vi "measure_once.vi"(8 "error in (no error)":errorcluster caption="エラー入力（エラーなし）", 9 "flux constant":T2, 10 "文字送り間隔 (100 ms)":i16=100, 11 "VISAリソース名":refnum<visa-resource-name>) -> (0 "error out":errorcluster caption="エラー出力", 2 "SQUID data":T1, 3 "VISAリソース名 （出力）":refnum<visa-resource-name>)   [LabVIEW 2017]
uses:
  controls/XYZ_Data.ctl
  controls/SQUID_data.ctl
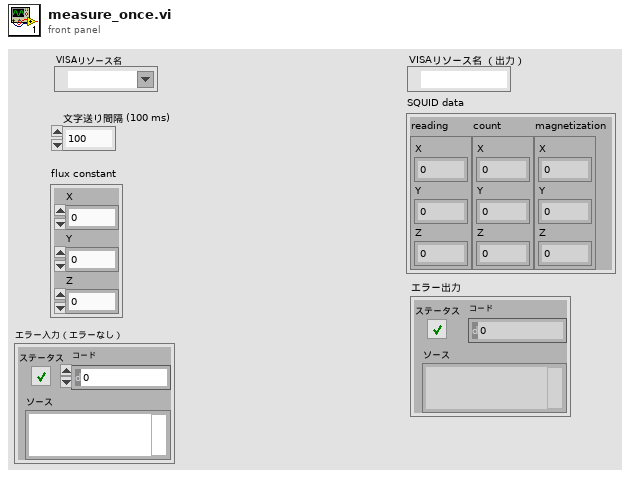
[diagram p1: front panel]
types:
  T1 = typedef "SQUID_data.ctl" = cluster{"reading":T2, "count":T2, "magnetization":T2}
  T2 = typedef "XYZ_Data.ctl" = cluster{"X":dbl, "Y":dbl, "Z":dbl}
  T3 = cluster{"読み取り":string, "読み取り":string, "読み取り":string}
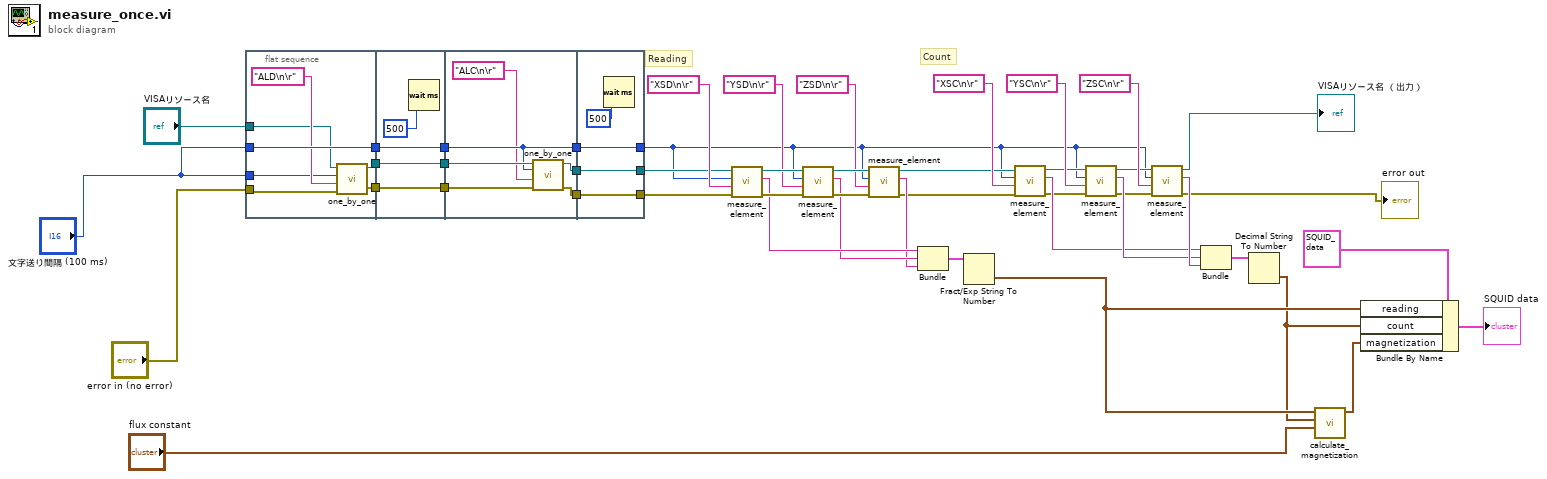
[diagram p0: block diagram]
diagram:
  # "Count"
  # "Reading"
  n1 = flat-sequence {
    tunnel: "文字送り間隔 (100 ms)" -> [w53]
    tunnel: [w48] -> w15
    tunnel: [w53] -> w14
    tunnel: [w49] -> w13
    tunnel: "文字送り間隔 (100 ms)" -> [w51]
    tunnel: "VISAリソース名" -> [w50]
    tunnel: "error in (no error)" -> [w47]
    tunnel: [w57] -> w18
    tunnel: [w55] -> w17
    tunnel: [w56] -> w16
    tunnel: w15 -> [w57]
    tunnel: w14 -> [w55]
    tunnel: w13 -> [w56]
    tunnel: w18 -> [w63]
    tunnel: w17 -> [w58]
    tunnel: w16 -> [w62]
    tunnel: [w61] -> w10
    tunnel: [w59] -> w9
    tunnel: [w58] -> w8
    tunnel: [w66] -> w19
    tunnel: [w67] -> w20
    tunnel: w10 -> [w67]
    tunnel: w9 -> [w66]
    tunnel: [w65] -> _
    tunnel: w8 -> [w65]
    frame #0 {
      n2 = call "one_by_one.vi"("error in (no error)"=w47, "入力文字"="ALD\n\r", "待機 (200ms)"=w51, "VISAリソース名"=w50) -> ("error out"=w49:errorcluster, "VISAリソース名出力"=w48:refnum<visa-resource-name>)  [unwired: 6 in]
    }
    frame #1 {
      n3 = Wait (ms)(milliseconds to wait=500) -> ()  [unwired: 1 out]
    }
    frame #2 {
      n4 = call "one_by_one.vi"("error in (no error)"=w62, "入力文字"="ALC\n\r", "待機 (200ms)"=w58, "VISAリソース名"=w63) -> ("error out"=w61:errorcluster, "VISAリソース名出力"=w59:refnum<visa-resource-name>)  [unwired: 6 in]
    }
    frame #3 {
      n5 = Wait (ms)(milliseconds to wait=500) -> ()  [unwired: 1 out]
    }
  }
  n6 = call "measure_element.vi"("error in (no error)"=w20, "コマンド"="XSD\n\r", "文字送り間隔 (200 ms)"="文字送り間隔 (100 ms)", "VISAリソース名"=w19) -> ("error out"=w44:errorcluster, "読み取り"=w39:string, "VISAリソース名 （出力）"=w45:refnum<visa-resource-name>)  [unwired: 5 in]
  n7 = call "measure_element.vi"("error in (no error)"=w44, "コマンド"="YSD\n\r", "文字送り間隔 (200 ms)"="文字送り間隔 (100 ms)", "VISAリソース名"=w45) -> ("error out"=w42:errorcluster, "読み取り"=w38:string, "VISAリソース名 （出力）"=w43:refnum<visa-resource-name>)  [unwired: 5 in]
  n8 = call "measure_element.vi"("error in (no error)"=w42, "コマンド"="ZSD\n\r", "文字送り間隔 (200 ms)"="文字送り間隔 (100 ms)", "VISAリソース名"=w43) -> ("error out"=w25:errorcluster, "読み取り"=w37:string, "VISAリソース名 （出力）"=w26:refnum<visa-resource-name>)  [unwired: 5 in]
  n9 = Bundle("読み取り"=w39, "読み取り"=w38, "読み取り"=w37) -> (w24:T3)  [unwired: 1 in]
  n10 = Fract/Exp String To Number(string=w24) -> (number=w4:cluster{"読み取り":dbl, "読み取り":dbl, "読み取り":dbl})  [unwired: 3 in, 1 out]
  n11 = call "measure_element.vi"("error in (no error)"=w25, "コマンド"="XSC\n\r", "文字送り間隔 (200 ms)"="文字送り間隔 (100 ms)", "VISAリソース名"=w26) -> ("error out"=w29:errorcluster, "読み取り"=w34:string, "VISAリソース名 （出力）"=w28:refnum<visa-resource-name>)  [unwired: 5 in]
  n12 = call "measure_element.vi"("error in (no error)"=w29, "コマンド"="YSC\n\r", "文字送り間隔 (200 ms)"="文字送り間隔 (100 ms)", "VISAリソース名"=w28) -> ("error out"=w31:errorcluster, "読み取り"=w35:string, "VISAリソース名 （出力）"=w30:refnum<visa-resource-name>)  [unwired: 5 in]
  n13 = call "measure_element.vi"("error in (no error)"=w31, "コマンド"="ZSC\n\r", "文字送り間隔 (200 ms)"="文字送り間隔 (100 ms)", "VISAリソース名"=w30) -> ("error out"=→"error out":errorcluster, "読み取り"=w36:string, "VISAリソース名 （出力）"=→"VISAリソース名 （出力）":refnum<visa-resource-name>)  [unwired: 5 in]
  n14 = Bundle("読み取り"=w34, "読み取り"=w35, "読み取り"=w36) -> (w23:T3)  [unwired: 1 in]
  n15 = Decimal String To Number(string=w23) -> (number=w3:cluster{"読み取り":i32, "読み取り":i32, "読み取り":i32})  [unwired: 2 in, 1 out]
  n16 = call "calculate_magnetization.vi"("Flux constant"="flux constant", "Count"=w3, "Reading"=w4) -> ("magnetization"=w2:T2)  [unwired: 8 in]
  n17 = Bundle By Name(cluster=T1 {"reading"={"X"=0.0, "Y"=0.0, "Z"=0.0}, "count"={"X"=0.0, "Y"=0.0, "Z"=0.0}, "magnetization"={"X"=0.0, "Y"=0.0, "Z"=0.0}} ("SQUID data"), "reading"=w4, "count"=w3, "magnetization"=w2) -> (→"SQUID data":T1)
